vi "StopProcesses.vi"(8 "error in (no error)":errorcluster, 9 "timeout in ms (-1)":i32=-1, 11 "SMO":refnum<class "SMO.lvclass">) -> (0 "error out":errorcluster, 3 "SMO out":refnum<class "SMO.lvclass">)   [LabVIEW 2019, in "SMO.lvclass"]
doc: "Stops all processes in the JKI SMO.\n\n---------------------------------------------------------------\nJKI State Machine Objects™\nhttp://jki.net/state-machine-objects/\nCopyright (C) 2005-2015, JKI <info@jki.net>\nALL RIGHTS RESERVEDJKI State Machine Objects (SMO) 1.3.0.56\nJKI - JKI\nCopyright (c) 2017, JKI"
uses:
  SMO.lvclass
  SMO.lvclass/SMO.ctl
panel:
  # "For instructions on how to use the JKI State Machine Objects, examples and video tutorials, visit:\nhttp://jki.net/state-machine-objects/\n\nJKI State Machine Objects™\nhttp://jki.net/state-machine-objects/\nCopyright (C) 2005-2015, JKI <info@jki.net>\nALL RIGHTS RESERVED"
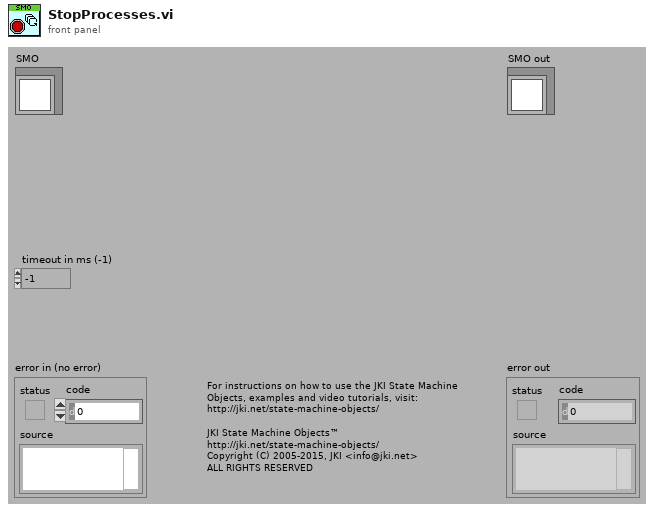
[diagram p1: front panel]
types:
  T1 = typedef "SMO.lvclass/Process Error Notification--Cluster.ctl" = cluster{"error":errorcluster}
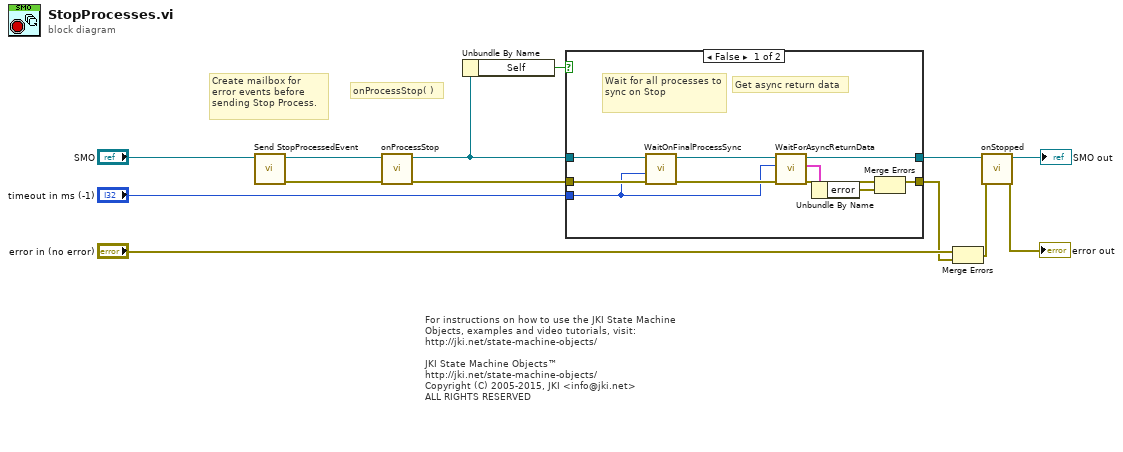
[diagram p0: block diagram]
diagram:
  # "onProcessStop( )"
  # "Create mailbox for\nerror events before\nsending Stop Process."
  # "For instructions on how to use the JKI State Machine Objects, examples and video tutorials, visit:\nhttp://jki.net/state-machine-objects/\n\nJKI State Machine Objects™\nhttp://jki.net/state-machine-objects/\nCopyright (C) 2005-2015, JKI <info@jki.net>\nALL RIGHTS RESERVED"
  n1 = call "Send StopProcessedEvent.vi"("SMO"="SMO") -> ("error out"=w12:errorcluster, "SMO out"=w10:refnum<class "SMO.lvclass">)  [unwired: 9 in]
  n2 = call-dynamic "onProcessStop.vi"("error in (no error)"=w12, "SMO"=w10) -> ("error out"=w11:errorcluster, "SMO out"=w1:refnum<class "SMO.lvclass">)  [unwired: 8 in]
  n3 = Unbundle By Name(w1) -> ("Self"=w3:bool)
  n4 = case shown="False" w3 {
    tunnel: w11 -> [w20 w24]
    tunnel: w1 -> [w19 w25]
    tunnel: [w18 w25] -> w7
    tunnel: "timeout in ms (-1)" -> [w17 _]
    tunnel: [w14 w24] -> w4
    frame False {
      # "Get async return data"
      # "Wait for all processes to sync on Stop"
      n5 = call "WaitOnFinalProcessSync.vi"("error in (no error)"=w20, "timeout in ms (-1)"=w17, "SMO"=w19) -> ("error out"=w21:errorcluster, "SMO out"=w22:refnum<class "SMO.lvclass">)  [unwired: 7 in]
      n6 = call "WaitForAsyncReturnData.vi"("error in (no error)"=w21, "timeout in ms (-1)"=w17, "SMO"=w22) -> ("error out"=w15:errorcluster, "Process Notification"=w23:T1, "SMO out"=w18:refnum<class "SMO.lvclass">)  [unwired: 6 in]
      n7 = Unbundle By Name(w23) -> ("error"=w16:errorcluster)
      n8 = Merge Errors(w15, w16) -> (w14:errorcluster)
    }
    frame True {
    }
  }
  n9 = Merge Errors("error in (no error)", w4) -> (w9:errorcluster)
  n10 = call-dynamic "onStopped.vi"("error in (no error)"=w9, "SMO"=w7) -> ("error out"=→"error out":errorcluster, "SMO out"=→"SMO out":refnum<class "SMO.lvclass">)  [unwired: 8 in]
